vi "FileSendResponse_Create.vi"(7 "Header":T3, 8 "error in (no error)":errorcluster, 9 "ResponseError":errorcluster, 10 "FileSendResponse":T1, 11 "IRoutingSource":T2) -> (0 "error out":errorcluster, 3 "Message":T5)   [LabVIEW 2017]
uses:
  <vilib>/addons/InsightCM/MessageBus/Base/controls/Message.ctl
  <vilib>/addons/InsightCM/MessageBus/Base/controls/MessageHeader.ctl
  <vilib>/addons/InsightCM/MessageBus/Base/controls/KeyValuePair.ctl
  <vilib>/addons/InsightCM/MessageBus/Base/controls/IRoutingSource.ctl
  <vilib>/addons/InsightCM/MessageBus/MessageLibrary/FileIngestion/controls/FileSendResponseBody.ctl
  <vilib>/addons/InsightCM/MessageBus/Base/controls/MessageClassType.ctl
  <vilib>/addons/InsightCM/Utilities/PropertyHelpers/PropertyHelpers.lvlib
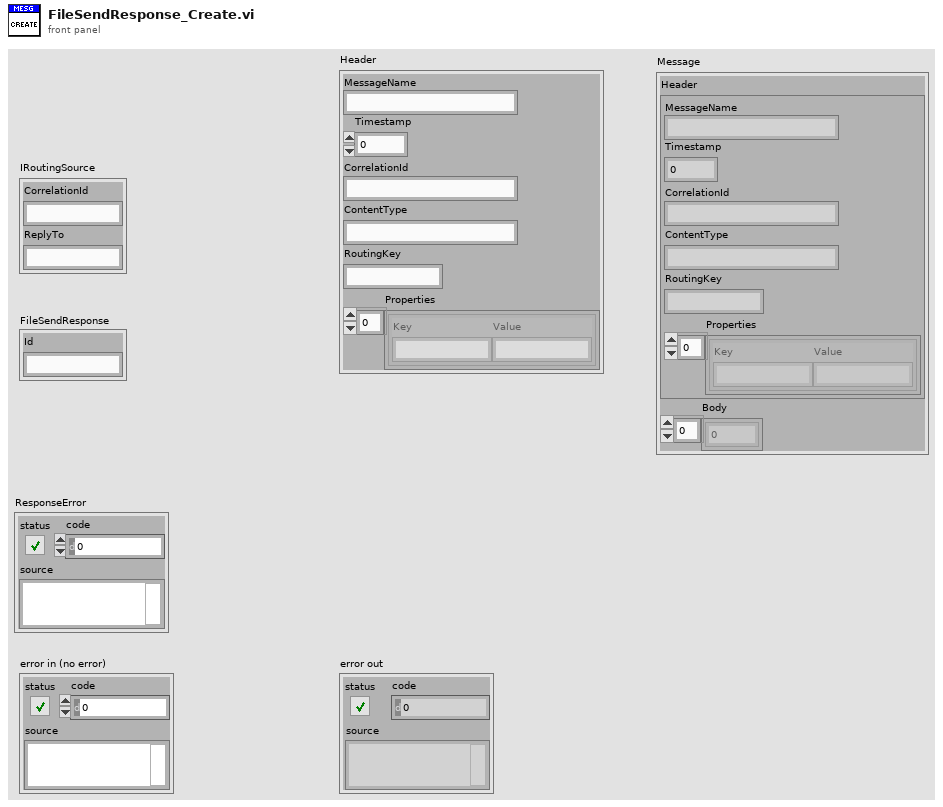
[diagram p1: front panel]
types:
  T1 = typedef "FileSendResponseBody.ctl" = cluster{"Id":string}
  T2 = typedef "IRoutingSource.ctl" = cluster{"CorrelationId":string, "ReplyTo":string}
  T3 = typedef "MessageHeader.ctl" = cluster{"MessageName":string, "Timestamp":i64, "CorrelationId":string, "ContentType":string, "RoutingKey":string, "Properties":T4[]}
  T4 = typedef "KeyValuePair.ctl" = cluster{"Key":string, "Value":string}
  T5 = typedef "Message.ctl" = cluster{"Header":T3, "Body":u8[]}
  T6 = typedef "MessageClassType.ctl" = enum16{"Request", "Response", "Broadcast", "RoutedMessage"}
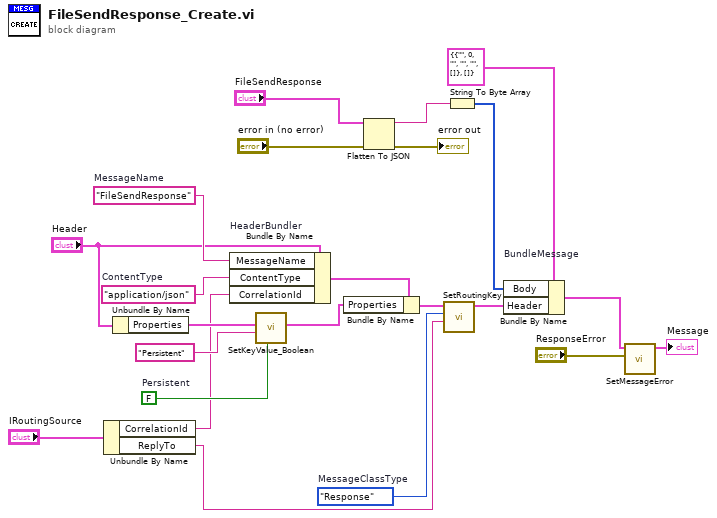
[diagram p0: block diagram]
diagram:
  w19 = MessageClassType."Response"  # MessageClassType
  w14 = FALSE  # Persistent
  w20 = "FileSendResponse"  # MessageName
  w17 = "application/json"  # ContentType
  n1 = Unbundle By Name("IRoutingSource") -> ("CorrelationId"=w4:string, "ReplyTo"=w3:string)
  n2 = Unbundle By Name("Header") -> ("Properties"=w16:T4[])
  n3 = Bundle By Name "HeaderBundler"(cluster="Header", "MessageName"=w20, "ContentType"=w17, "CorrelationId"=w4) -> (w11:T3)
  n4 = call <vilib>:"SetKeyValue_Boolean.vi"("value"=w14, "key"="Persistent" ("Key"), "key value pairs"=w16) -> ("key value pairs out"=w10:T4[])  [unwired: 8 in]
  n5 = Bundle By Name(cluster=w11, "Properties"=w10) -> (w12:T3)
  n6 = Flatten To JSON(anything="FileSendResponse", error in (no error)="error in (no error)") -> (JSON string=w2:string, 11:→"error out":errorcluster)  [unwired: 1 in]
  n7 = call <vilib>:"SetRoutingKey.vi"("SendTo"=w3, "MessageClassType"=w19, "Message Header in"=w12) -> ("Message Header out"=w13:T3)  [unwired: 8 in]
  n8 = String To Byte Array(string=w2) -> (unsigned byte array=w22:u8[])
  n9 = Bundle By Name "BundleMessage"(cluster=T5 {"Header"={"MessageName"="", "Timestamp"=0, "CorrelationId"="", "ContentType"="", "RoutingKey"="", "Properties"=[]}, "Body"=[]} ("Message"), "Body"=w22, "Header"=w13) -> (w8:T5)
  n10 = call <vilib>:"SetMessageError.vi"("error"="ResponseError", "message in"=w8) -> ("message out"=→"Message":T5)  [unwired: 9 in]
